vi "Create Attribute.vi"(8 "error in (no error)":errorcluster, 9 "Value":string, 10 "Name":string="testsuite", 11 "Element in":refnum<k20>) -> (0 "error out":errorcluster, 3 "Element out":refnum<k20>)   [LabVIEW 2013, in "XML.lvlib"]
doc: "Adds an attribute to an element. The caller is responsible for cleaning up references."
uses:
  XML.lvlib
  <resource>/objmgr/DOMUserDefRef.rc
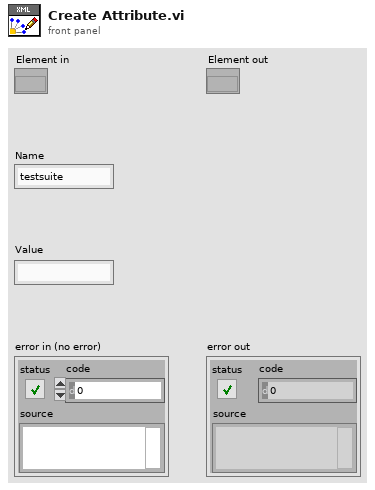
[diagram p1: front panel]
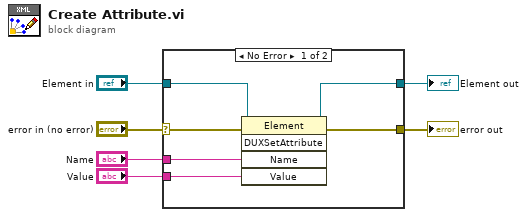
[diagram p0: block diagram]
diagram:
  n1 = case shown="No Error" "error in (no error)" {
    selector: "error in (no error)" -> [w8 w14]
    tunnel: "Element in" -> [w11 w13]
    tunnel: [w10 w13] -> w5
    tunnel: "Name" -> [w12 _]
    tunnel: [w9 w14] -> w3
    tunnel: "Value" -> [w7 _]
    frame No Error {
      n2 = invoke class="Element" method="DUXSetAttribute"(reference=w11, error in=w8, "Name"=w12, "Value"=w7) -> (reference out=w10:refnum<k20>, error out=w9:errorcluster)  [unwired: 1 in, 3 out]
    }
    frame Error {
    }
  }
  "Element out" <- w5
  "error out" <- w3
